vi "MWriteRS232.vi"(8 "P3":dbl, 9 "P2":dbl, 10 "P1":dbl, 11 "LAUDA":dbl=22.0) -> ()   [LabVIEW 2015]
uses:
  BERTTA.dll
panel:
  in  "dev4":i32=2
  in  "port4":i32=14
  in  "dev3":i32=2
  in  "port3":i32=15
  in  "dev2":i32=2
  in  "port2":i32=16
  in  "dev1":i32=1
  in  "port1":i32=9
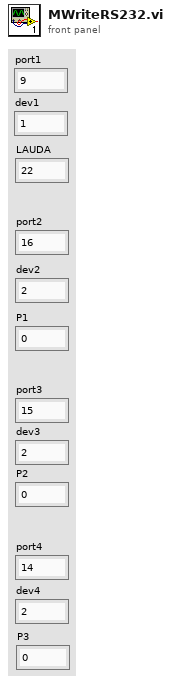
[diagram p1: front panel]
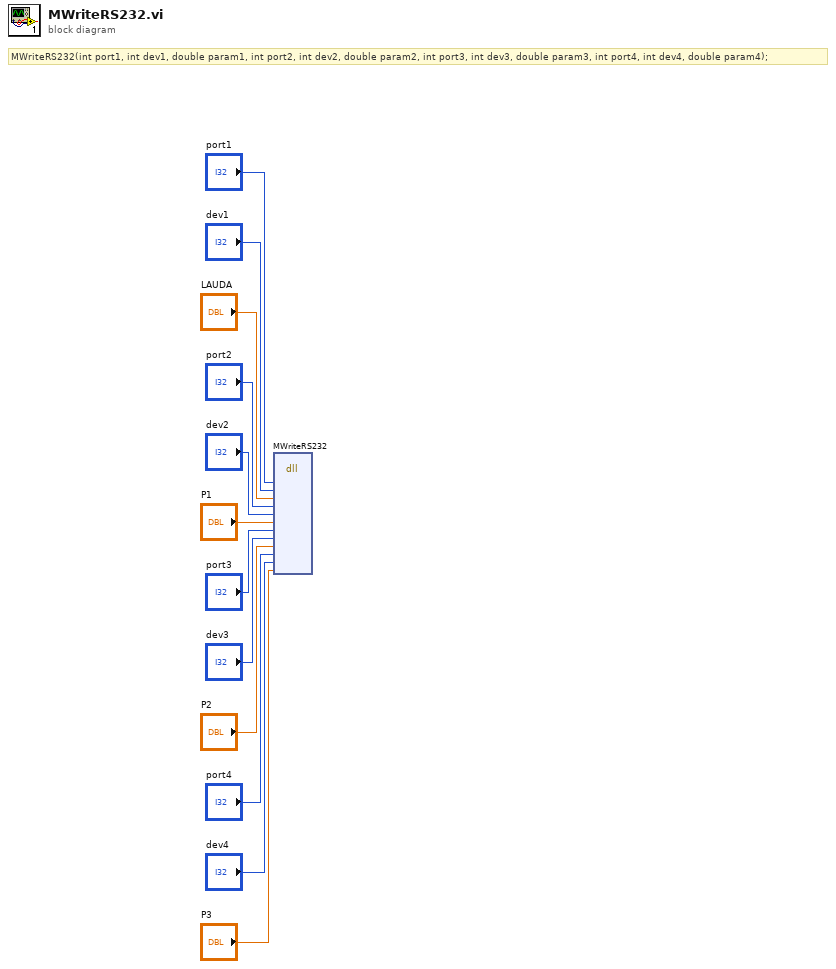
[diagram p0: block diagram]
diagram:
  # "MWriteRS232(int port1, int dev1, double param1, int port2, int dev2, double param2, int port3, int dev3, double param3, int port4, int dev4, double param4);"
  n1 = dll-call lib="C:/Users/shresplab/OneDrive - Kemira Oyj/Documents/Visual Studio 2017/Projects/Bertta/BERTTA/x64/Debug/BERTTA.dll" fn="MWriteRS232"("port1"="port1", "dev1"="dev1", "param1"="LAUDA", "port2"="port2", "dev2"="dev2", "param2"="P1", "port3"="port3", "dev3"="dev3", "param3"="P2", "port4"="port4", "dev4"="dev4", "param4"="P3") -> ()  [unwired: 16 in, 2 out]
